vi "1L03-insere_0_tab1D.vi"(1 "t":dbl[](array[numeric])) -> (0 "t":dbl[](array[numeric]))   [LabVIEW 2010, in "lv_01.lvlib"]
doc: "Si le tableau en entrée ne contient pas de 0 à l'indice 0, alors on l'ajoute."
uses:
  lv_01.lvlib
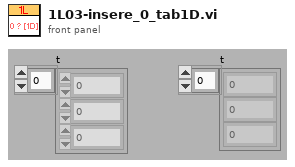
[diagram p1: front panel]
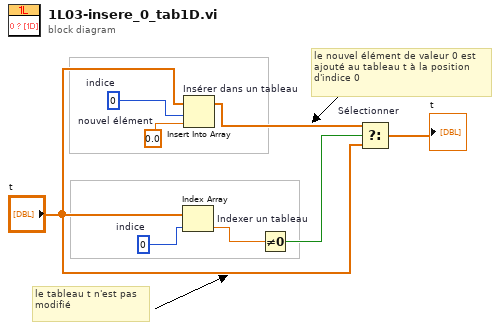
[diagram p0: block diagram]
diagram:
  w7 = 0.0  # nouvel élément
  w6 = 0  # indice
  w8 = 0  # indice
  # "le tableau t n'est pas modifié"
  # "le nouvel élément de valeur 0 est ajouté au tableau t à la position d'indice 0"
  n1 = Index Array "Indexer un tableau"(array="t", index=w8) -> (element=w2:dbl)
  n2 = Insert Into Array "Insérer dans un tableau"(array="t", index=w6, new element=w7) -> (w5:dbl[])
  n3 = Not Equal To 0?(x=w2) -> (x != 0?=w1:bool)
  n4 = Select "Sélectionner"(t=w5, s=w1, f="t") -> (s? t:f=→"t":dbl[])
